vi "FG QNodeList.vi"(1 "FG Action (Read)":T1, 2 "NodeList in":T2[](array[typedef])) -> (0 "NodeList out":T2[](array[typedef]))   [LabVIEW 2009]
uses:
  NodeRec.ctl
  ComponentRec.ctl
  ServiceRec.ctl
  cRIO/Functional Global Variables/Actions for FG's.ctl
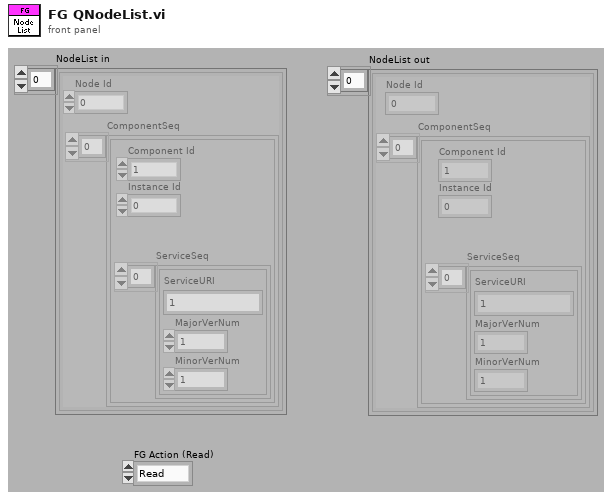
[diagram p1: front panel]
types:
  T1 = typedef "Actions for FG's.ctl" = enum16{"Read", "Write"}
  T2 = typedef "NodeRec.ctl" = cluster{"Node Id":u8, "ComponentSeq":T3[]}
  T3 = typedef "ComponentRec.ctl" = cluster{"Component Id":u8, "Instance Id":u8, "ServiceSeq":T4[]}
  T4 = typedef "ServiceRec.ctl" = cluster{"ServiceURI":string, "MajorVerNum":u8, "MinorVerNum":u8}
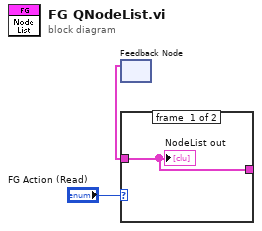
[diagram p0: block diagram]
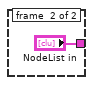
[diagram p2: hidden frame]
diagram:
  n1 = feedback #1() -> (w1:T2[])  [unwired: 1 in]
  n2 = case shown="\"Write\"" "FG Action (Read)" {
    tunnel: [w4 "NodeList in"] -> w3
    tunnel: w1 -> [w4 _]
    frame #0 {
      "NodeList out" <- w4
    }
    frame #1 {
    }
  }
